vi "Data Packaging Loop.vi"(6 "Message Queues":T1 caption="消息队列", 7 "channel info array":cluster{"Module":string, "Channel":string}[](array[cluster]) caption="通道信息", 8 "error in (no error)":errorcluster caption="错误输入（无错误）", 9 "sampling period (s)":dbl caption="采用周期 (s)", 10 "timestamp":timestamp caption="时间标识", 11 "data queue":refnum<queue> caption="数据队列") -> (0 "error out":errorcluster caption="错误输出")   [LabVIEW 2015]
uses:
  Support VIs/Message Queue/All Real-Time Message Queues.ctl
  Support VIs/Message Queue/Message Cluster.ctl
  Globals/Global - All RT Loop Stop.vi
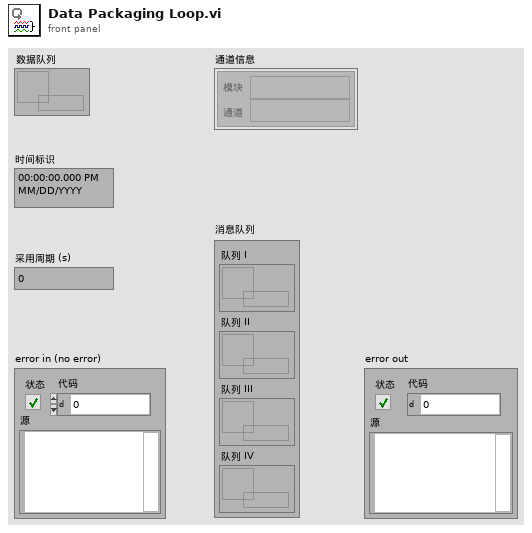
[diagram p1: front panel]
types:
  T1 = typedef "Message Queue.lvlib/All Real-Time Message Queues.ctl" = cluster{"Queue I":refnum<queue>, "Queue II":refnum<queue>, "Queue III":refnum<queue>, "Queue IV":refnum<queue>}
  T2 = enum16{"Initialize", "Acquire Data", "Create Waveform", "Send Waveform"}
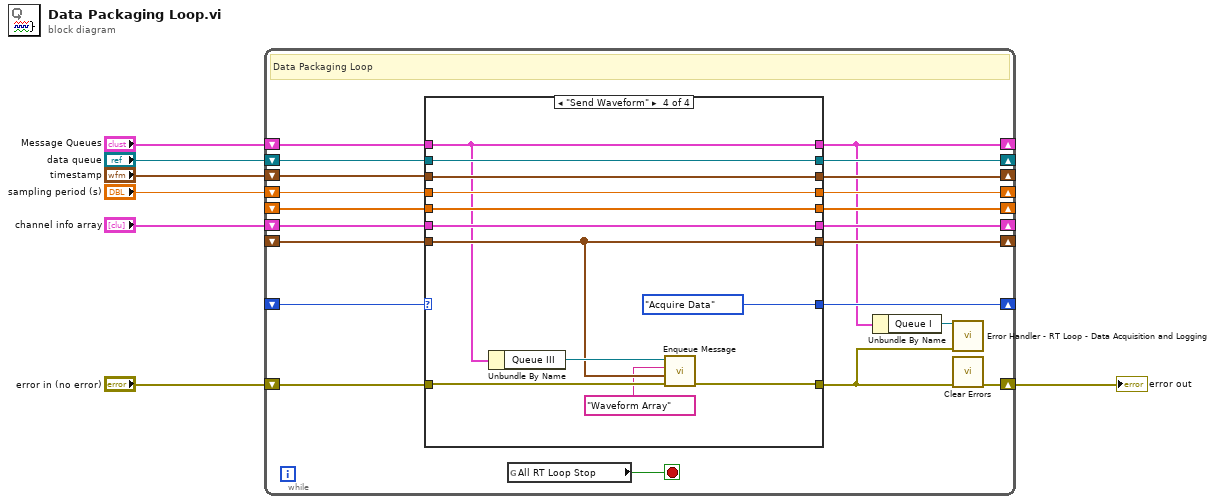
[diagram p0: block diagram]
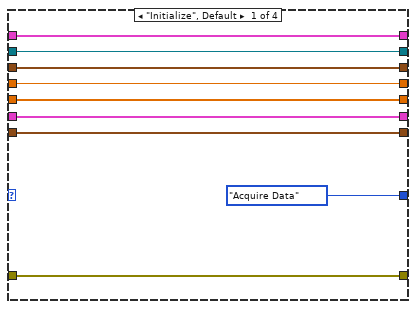
[diagram p2: hidden frame]
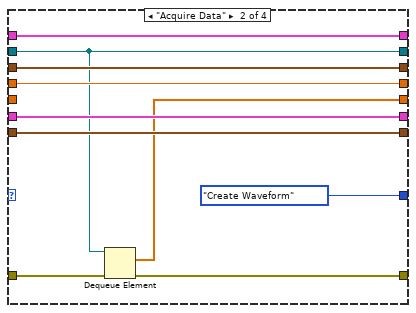
[diagram p3: hidden frame]
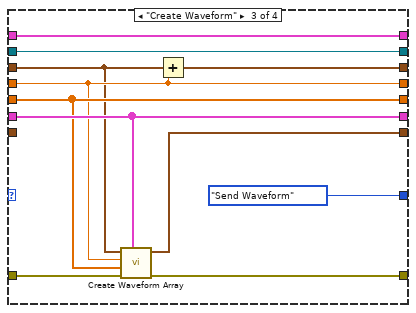
[diagram p4: hidden frame]
diagram:
  n1 = while {
    shift-right: [w28] -> _
    shift-left: "timestamp" -> [w27]
    shift-right: [w21] -> _
    shift-left: _ -> [w22]
    shift-right: [w8] -> _
    shift-left: "Message Queues" -> [w20]
    shift-right: [w19] -> _
    shift-left: _ -> [w18]
    shift-right: [w17] -> w1
    shift-left: "error in (no error)" -> [w25]
    shift-right: [w15] -> _
    shift-left: "data queue" -> [w26]
    shift-right: [w10] -> _
    shift-left: "channel info array" -> [w23]
    shift-right: [w14] -> _
    shift-left: _ -> [w13]
    shift-right: [w9] -> _
    shift-left: "sampling period (s)" -> [w11]
    stop <- w24 stop-if-true
    # "Data Packaging Loop"
    n2 = case shown="\"Send Waveform\"" w22 {
      tunnel: [w32 w43 w49 w64] -> w28
      tunnel: w27 -> [w32 w43 w48 w64]
      tunnel: w23 -> [w33 w41 w52 w65]
      tunnel: w26 -> [w34 w38 w53 w66]
      tunnel: w25 -> [w37 w46 w58 w69]
      tunnel: [w37 w47 w55 w68] -> w16
      tunnel: [T2."Acquire Data" T2."Create Waveform" T2."Send Waveform" T2."Acquire Data"] -> w21
      tunnel: w20 -> [w35 w44 w54 w60]
      tunnel: [w35 w44 w54 w60] -> w8
      tunnel: [w30 w39 w51 w62] -> w19
      tunnel: w18 -> [w30 _ w51 w62]
      tunnel: [w34 w38 w53 w66] -> w15
      tunnel: [w29 w40 w56 w61] -> w14
      tunnel: w13 -> [w29 w40 _ w61]
      tunnel: w11 -> [w31 w42 w50 w63]
      tunnel: [w33 w41 w52 w65] -> w10
      tunnel: [w31 w42 w50 w63] -> w9
      frame "Initialize", Default {
      }
      frame "Acquire Data" {
        n3 = Dequeue Element(queue=w38, error in (no error)=w46) -> (element=w39:dbl[], error out=w47:errorcluster)  [unwired: 1 in, 2 out]
      }
      frame "Create Waveform" {
        n4 = call "Create Waveform Array.vi"("channel info array"=w52, "error in (no error)"=w58, "samples to write"=w51, "sampling period (s)"=w50, "Timestamp"=w48) -> ("error out"=w55:errorcluster, "Waveform Array"=w56:waveform(dbl)[])  [unwired: 5 in]
        n5 = Add(x=w48, y=w50) -> (x+y=w49:timestamp)
      }
      frame "Send Waveform" {
        n6 = Unbundle By Name(w60) -> ("Queue III"=w67:refnum<queue>)
        n7 = call "Enqueue Message.vi"("error in (no error)"=w69, "Message Data"=w61, "Message"="Waveform Array", "Message Queue"=w67) -> ("error out"=w68:errorcluster)  [unwired: 6 in, 1 out]
      }
    }
    n8 = global read "Global - All RT Loop Stop.vi" "All RT Loop Stop"() -> (w24:bool)
    n9 = Unbundle By Name(w8) -> ("Queue I"=w12:refnum<queue>)
    n10 = call "Error Handler - RT Loop - Data Acquisition and Logging.vi"("error in (no error)"=w16, "Message Queue"=w12) -> ()  [unwired: 9 in, 1 out]
    n11 = call <vilib>:"Clear Errors.vi"("error in (no error)"=w16) -> ("error out"=w17:errorcluster)  [unwired: 5 in, 1 out]
  }
  "error out" <- w1
